vi "Waveform to FPGA.vi"(0 "Write Frame Galvo signal?":bool, 1 "max addr":u32=1000, 2 "Write DRAM enable?":bool, 3 "Total elements":u32=512000) -> (7 "Write DRAM done?":bool, 9 "Frame Galvo signal write done?":bool)   [LabVIEW 2015]
uses:
  <vilib>/Platform/TimedLoop/XDataNode/timing_clust.ctl
  <vilib>/Platform/TimedLoop/XDataNode/nitl_modes.ctl
  <vilib>/Platform/TimedLoop/XDataNode/wakeup.ctl
  OpenScan Labview code_20170126/DRAM data index.ctl
  <vilib>/rvi/Emulation/niFpgaSctlEmulationGetInTimedLoop.vi
  <vilib>/rvi/Emulation/niFpgaEmulationReportErrorSimple.vi
  <vilib>/rvi/Emulation/niFpgaGetClockAttributes.vi
  <vilib>/rvi/Emulation/niFpgaCriticalErrorInLSC.vi
  Globals/Global_Sample per Frame.vi
  <vilib>/rvi/Emulation/niFpgaProcessEmulError.vi
  <vilib>/Platform/TimedLoop/XDataNode/XDataNode.xnode
  <vilib>/Platform/TimedLoop/XDataNode/XDNodeRunTimeDep.lvlib
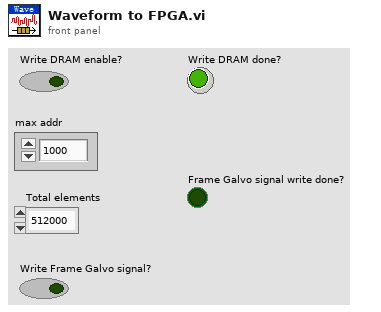
[diagram p1: front panel]
types:
  T1 = typedef "DRAM data index.ctl" = enum16{"Numeric 1", "Numeric 2", "Numeric 3", "Numeric 4", "Numeric 5", "Numeric 6", "Numeric 7", "Numeric 8", "Numeric 9", "Numeric 10", "Numeric 11", "Numeric 12", "Numeric 13", "Numeric 14", "Numeric 15", "Numeric 16"}
  T2 = cluster{"Numeric 1":u32, "Numeric 2":u32, "Numeric 3":u32, "Numeric 4":u32, "Numeric 5":u32, "Numeric 6":u32, "Numeric 7":u32, "Numeric 8":u32, "Numeric 9":u32, "Numeric 10":u32, "Numeric 11":u32, "Numeric 12":u32, "Numeric 13":u32, "Numeric 14":u32, "Numeric 15":u32, "Numeric 16":u32}
  T3 = typedef "XDNodeRunTimeDep.lvlib/timing_clust.ctl" = cluster{"Expected End [f-1]":u64, "Actual End [f-1]":u64, "Finished Late? [f-1]":bool, "Expected End [i-1]":u64, "Actual End [i-1]":u64, "Finished Late? [i-1]":bool, "Expected Start [i]":u64, "Actual Start [i]":u64, "Expected Start [f]":u64, "Actual Start [f]":u64, "Source Name":string, "Structure Name":string, "Period":i64, "Deadline":i64, "Offset":i64, "Start":i64, "Priority":i32, "Timeout":i32, "Mode":T4, "Wakeup Reason":T5, "Error":errorcluster, "Source Type":string, "Secondary Source Type":string, "Global End Time":u64, "Global Start Time":u64, "Frame Duration":u64, "Iteration Duration":u64, "Assigned CPU":i32, "I/O Scan Engine Mode":u32}
  T4 = typedef "XDNodeRunTimeDep.lvlib/nitl_modes.ctl" = enum32{"No Change", "Process missed periods, maintain original phase", "Discard missed periods, maintain original phase", "Process missed periods, ignore original phase", "Discard missed periods, ignore original phase"}
  T5 = typedef "XDNodeRunTimeDep.lvlib/wakeup.ctl" = enum32{"Normal", "Aborted", "Asynchronous wakeup", "Timing source error", "Timed loop error", "Timeout"}
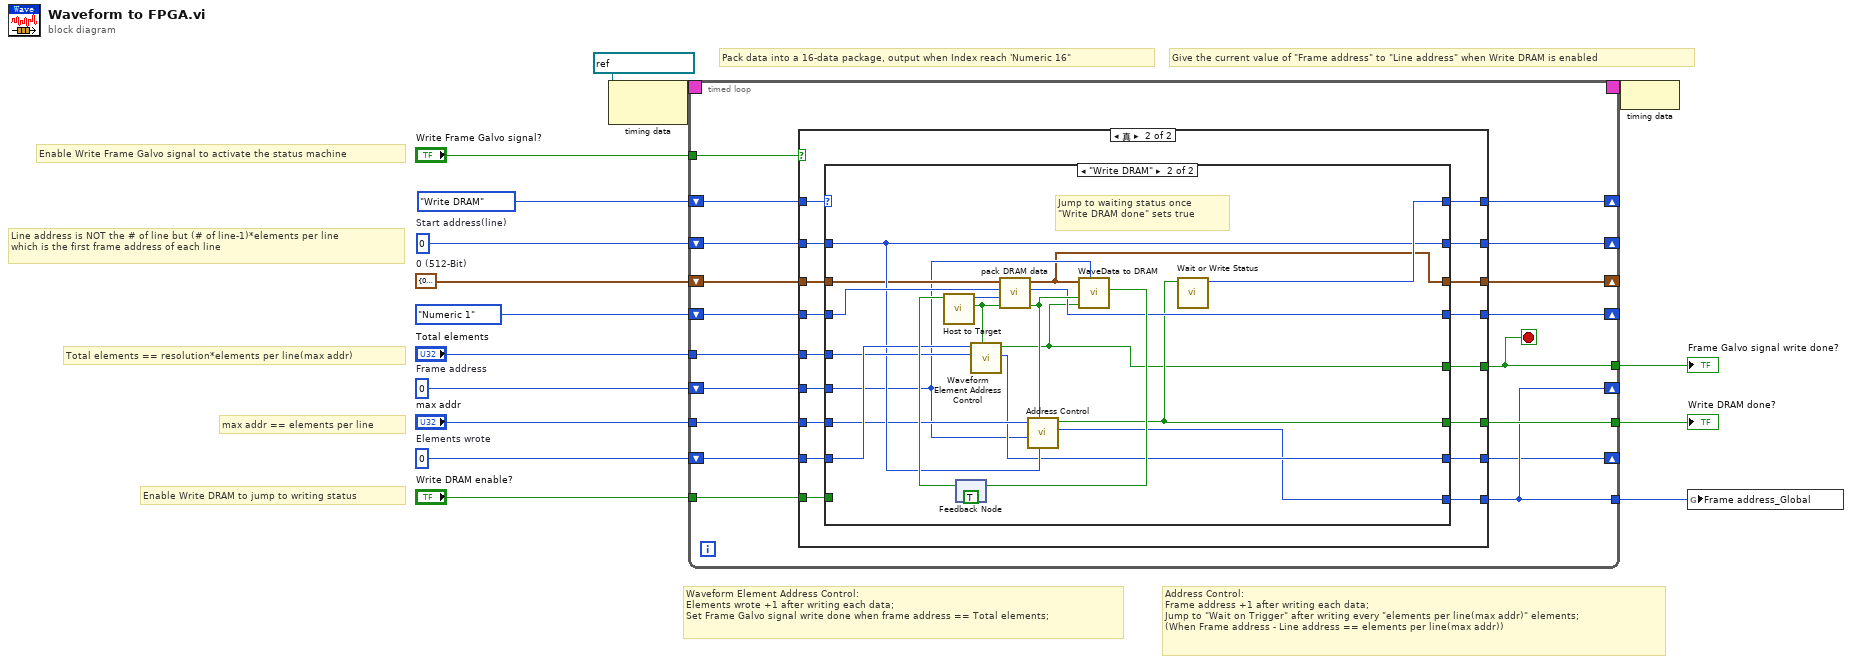
[diagram p0: block diagram]
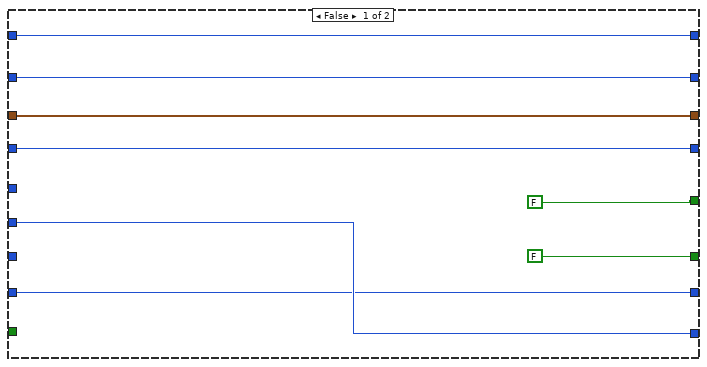
[diagram p2: hidden frame]
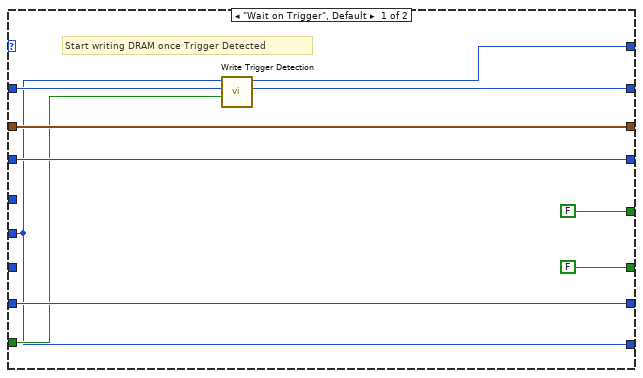
[diagram p3: hidden frame]
diagram:
  w3 = u32 0  # Elements wrote
  w5 = T2 {"Numeric 1"=0, "Numeric 2"=0, "Numeric 3"=0, "Numeric 4"=0, "Numeric 5"=0, "Numeric 6"=0, "Numeric 7"=0, "Numeric 8"=0, "Numeric 9"=0, "Numeric 10"=0, "Numeric 11"=0, "Numeric 12"=0, "Numeric 13"=0, "Numeric 14"=0, "Numeric 15"=0, "Numeric 16"=0}  # 0 (512-Bit)
  w13 = u32 0  # Start address(line)
  w14 = u32 0  # Frame address
  # "Give the current value of \"Frame address\" to \"Line address\" when Write DRAM is enabled"
  # "Pack data into a 16-data package, output when Index reach 'Numeric 16\""
  # "Address Control:\nFrame address +1 after writing each data;\nJump to \"Wait on Trigger\" after writing every \"elements per line(max addr)\" elements;\n(When Frame address - Line address == elements per line(max addr))"
  # "Waveform Element Address Control:\nElements wrote +1 after writing each data;\nSet Frame Galvo signal write done when frame address == Total elements;"
  # "max addr == elements per line"
  # "Total elements == resolution*elements per line(max addr)"
  # "Line address is NOT the # of line but (# of line-1)*elements per line\nwhich is the first frame address of each line"
  # "Enable Write DRAM to jump to writing status"
  # "Enable Write Frame Galvo signal to activate the status machine"
  n1 = node-c288(refnum<k21> "DRAM Clock" ("Source Name")) -> (w16:T3)
  n2 = timed-loop {
    timing: w16 -> [_]
    timing-out: [_] -> w15
    shift-right: [w32] -> _
    shift-left: w13 -> [w34]
    shift-right: [w27] -> _
    shift-left: w14 -> [w33]
    tunnel: "Write Frame Galvo signal?" -> [w31]
    tunnel: "max addr" -> [w30]
    tunnel: [w29] -> w9
    tunnel: "Total elements" -> [w20]
    tunnel: [w19] -> w7
    tunnel: "Write DRAM enable?" -> [w28]
    tunnel: [w27] -> w2
    shift-right: [w26] -> _
    shift-left: w5 -> [w25]
    shift-right: [w23] -> _
    shift-left: DRAM_data_index."Numeric 1" ("Galvo index in") -> [w24]
    shift-right: [w21] -> _
    shift-left: w3 -> [w22]
    shift-right: [w17] -> _
    shift-left: enum16{"Wait on Trigger", "Write DRAM"}."Write DRAM" -> [w18]
    stop <- w19 stop-if-true
    n3 = case shown="真" w31 {
      tunnel: w33 -> [w42 w59]
      tunnel: w34 -> [w41 w58]
      tunnel: [w42 w57] -> w27
      tunnel: [w41 w56] -> w32
      tunnel: w30 -> [_ w55]
      tunnel: [FALSE w54] -> w29
      tunnel: w28 -> [_ w53]
      tunnel: w25 -> [w39 w51]
      tunnel: [w39 w52] -> w26
      tunnel: w24 -> [w38 w50]
      tunnel: [w38 w49] -> w23
      tunnel: w22 -> [w37 w48]
      tunnel: [w37 w47] -> w21
      tunnel: w20 -> [_ w46]
      tunnel: [FALSE w45] -> w19
      tunnel: w18 -> [w35 w44]
      tunnel: [w35 w43] -> w17
      frame False {
      }
      frame True {
        n4 = case shown="\"Write DRAM\"" w44 {
          tunnel: w59 -> [w61 w74]
          tunnel: [w61 w73] -> w57
          tunnel: w58 -> [w64 w80]
          tunnel: [w62 w80] -> w56
          tunnel: w55 -> [_ w79]
          tunnel: [FALSE w72] -> w54
          tunnel: w53 -> [w63 _]
          tunnel: w51 -> [w68 w78]
          tunnel: [w68 w71] -> w52
          tunnel: w50 -> [w67 w81]
          tunnel: [w67 w75] -> w49
          tunnel: w48 -> [w66 w83]
          tunnel: [w66 w77] -> w47
          tunnel: w46 -> [_ w82]
          tunnel: [FALSE w70] -> w45
          tunnel: [w60 w84] -> w43
          frame "Wait on Trigger", Default {
            # "Start writing DRAM once Trigger Detected"
            n5 = call "Write Trigger Detection.vi"("Write DRAM enable?"=w63, "Start address(line) in"=w64, "Start address(frame) in"=w61) -> ("Start address(line) out"=w62:u32, "Next Status"=w60:enum16{"Wait on Trigger", "Write DRAM"})  [unwired: 7 in]
          }
          frame "Write DRAM" {
            # "Jump to waiting status once\n\"Write DRAM done\" sets true"
            n6 = feedback #1(TRUE ("Ready for Input")) -> (w88:bool)
            n7 = call "Host to Target.vi"("Ready for Input"=w88) -> ("Output Valid"=w76:bool, "Data"=w87:u32)  [unwired: 9 in]
            n8 = call "Waveform Element Address Control.vi"("s"=w76, "Total elements"=w82, "Elements wrote in"=w83) -> ("Elements wrote out"=w77:u32, "Output Valid"=w70:bool)  [unwired: 7 in]
            n9 = call "pack DRAM data.vi"("input valid?"=w76, "data to be packed"=w87, "DRAM Index in"=w81, "packer in"=w78) -> ("output valid?"=w86:bool, "DRAM Index out"=w75:T1, "packer out"=w71:T2)  [unwired: 5 in]
            n10 = call "Address Control.vi"("Address(line)"=w80, "output valid?"=w86, "Address(frame) input in"=w74, "max addr"=w79) -> ("Address(frame) input out"=w73:u32, "input ready"=w72:bool)  [unwired: 6 in]
            n11 = call "WaveData to DRAM.vi"("Address(frame) input"=w74, "input valid? 2"=w70, "input valid?"=w86, "packer out"=w71) -> ("Input ready"=w85:bool)  [unwired: 7 in]
            n12 = feedback-in #1(w85) -> ()
            n13 = call "Wait or Write Status.vi"("reach end"=w72) -> ("Next Status"=w84:enum16{"Wait on Trigger", "Write DRAM"})  [unwired: 10 in]
          }
        }
      }
    }
  }
  "Write DRAM done?" <- w9
  "Frame Galvo signal write done?" <- w7
  n14 = node-c288(w15) -> ()
  n15 = global write "Global_Sample per Frame.vi" "Frame address_Global"(w2) -> ()
